vi "re_DataLog Write Number.vi"(0 "number":dbl format="%#_7g", 5 "time (current)":dbl=nan format="%<%H:%M:%S%2u\n%Y/%m/%d>T", 7 "tag":string, 9 "tag index in (use tag)":i32=-1, 11 "error in (no error)":errorcluster) -> (10 "tag index out":i32, 15 "error out":errorcluster)   [LabVIEW 2012]
doc: "Writes a number value to a tag. The current time is used as timestamp if no custom time is wired. The value is checked against any limit meta tags and coerced to any max/min meta tags. The current database must be live."
uses:
  typedefs/t_DataLog Tag Meta Tags Methods.ctl
  typedefs/clusters/t_DataLog Point.ctl
  typedefs/t_DataLog Tag Hash Methods.ctl
  luaview/typedefs/t_LuaVIEW Task List Methods.ctl
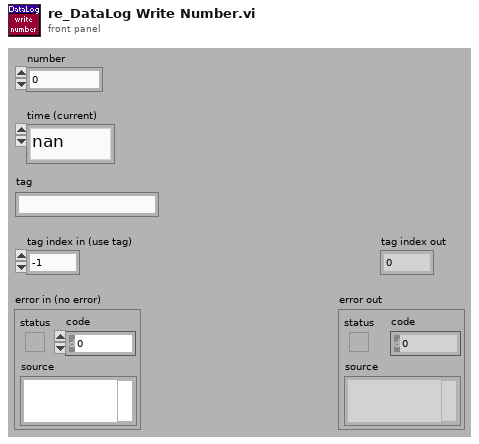
[diagram p1: front panel]
types:
  T1 = typedef "t_DataLog Point.ctl" = cluster{"time":dbl, "value":dbl}
  T2 = typedef "t_DataLog Tag Meta Tags Methods.ctl" = enum16{"initialize", "apply and write", "get exceeded", "get metas", "cleanup"}
  T3 = typedef "t_LuaVIEW Task List Methods.ctl" = enum16{"clear list", "add", "test", "remove", "get ref", "get task info", "get list", "get script info", "ongoing?", "resume", "pause", "stop", "confirm", "message"}
  T4 = typedef "t_DataLog Tag Hash Methods.ctl" = enum16{"initialize", "add tag", "index tag", "lookup", "#tags", "cleanup", "write recovery", "read recovery", "delete recovery"}
  T5 = typedef "et_DataLog Meta Tag Specifier.ctl" = enum32{"warn_lo", "warn_hi", "A_lo", "A_hi", "B_lo", "B_hi", "C_lo", "C_hi", "D_lo", "D_hi", "E_lo", "E_hi", "F_lo", "F_hi", "G_lo", "G_hi", "H_lo", "H_hi", "I_lo", "I_hi", "J_lo", "J_hi", "K_lo", "K_hi", "L_lo", "L_hi", "M_lo", "M_hi", "N_lo", "N_hi", "min", "max", "not a meta"}
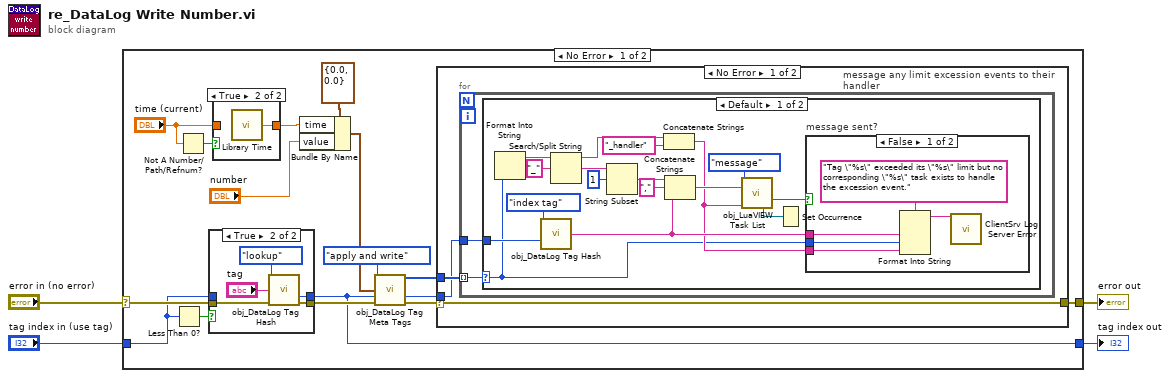
[diagram p0: block diagram]
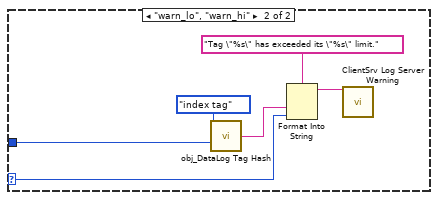
[diagram p4: hidden frame]
diagram:
  n1 = case shown="No Error" "error in (no error)" {
    selector: "error in (no error)" -> [w20 w65]
    tunnel: [w15 w65] -> w4
    tunnel: "tag index in (use tag)" -> [w6 w64]
    tunnel: [w5 w64] -> w1
    frame No Error {
      n2 = Less Than 0?(x=w6) -> (x < 0?=w19:bool)
      n3 = Not A Number/Path/Refnum?(number/path/refnum="time (current)") -> (NaN/Path/Refnum?=w12:bool)
      n4 = case shown="True" w19 {
        tunnel: w20 -> [w58 w63]
        tunnel: [w58 w61] -> w17
        tunnel: [w57 w60] -> w5
        tunnel: w6 -> [w57 _]
        frame False {
        }
        frame True {
          n5 = call "obj_DataLog Tag Hash.vi"("method"=t_DataLog_Tag_Hash_Methods."lookup", "tag in"="tag", "error in (no error)"=w63) -> ("tag index out"=w60:i32, "error out"=w61:errorcluster)  [unwired: 9 in, 2 out]
        }
      }
      n6 = case shown="True" w12 {
        tunnel: "time (current)" -> [w21 _]
        tunnel: [w21 w22] -> w10
        frame False {
        }
        frame True {
          n7 = call "Library Time.vi"() -> ("time"=w22:dbl)  [unwired: 1 in]
        }
      }
      n8 = Bundle By Name(cluster=T1 {"time"=0.0, "value"=0.0} ("point"), "time"=w10, "value"="number") -> (w7:T1)
      n9 = call "obj_DataLog Tag Meta Tags.vi"("method"=t_DataLog_Tag_Meta_Tags_Methods."apply and write", "point to write"=w7, "tag index in"=w5, "error in (no error)"=w17) -> ("limit events"=w14:T5[], "tag index dup"=w13:i32, "error out"=w16:errorcluster)  [unwired: 7 in, 2 out]
      n10 = case shown="No Error" w16 {
        selector: w16 -> [w23 w56]
        tunnel: [w23 w56] -> w15
        tunnel: w14 -> [w25 _]
        tunnel: w13 -> [w24 _]
        frame No Error {
          n11 = for "message any limit excession events to their handler" {
            tunnel: w25 -> [w26] mode=indexing
            tunnel: w24 -> [w27]
            n12 = case shown="Default" w26 {
              selector: w26 -> [w28 w51]
              tunnel: w27 -> [w35 w54]
              frame Default {
                n13 = Format Into String(w28) -> (resulting string=w44:string)  [unwired: 3 in, 1 out]
                n14 = call "obj_DataLog Tag Hash.vi"("method"=t_DataLog_Tag_Hash_Methods."index tag", "tag index in"=w35) -> ("tag out"=w31:string)  [unwired: 10 in, 3 out]
                n15 = Search/Split String(string=w44, search string/char (-)="_") -> (substring before match=w39:string, match + rest of string=w42:string)  [unwired: 1 in, 1 out]
                n16 = String Subset(string=w42, offset (0)=1) -> (substring=w40:string)  [unwired: 1 in]
                n17 = Concatenate Strings(w39, "_handler" ("string")) -> (w30:string)
                n18 = Concatenate Strings(w40, "," ("string"), w31) -> (w33:string)
                n19 = call "obj_LuaVIEW Task List.vi"("method"=t_LuaVIEW_Task_List_Methods."message", "message"=w33, "task identifier"=w30) -> ("set/ongoing"=w32:bool, "wakeup occurrence"=w29:refnum<k4>)  [unwired: 7 in, 4 out]
                n20 = Set Occurrence(w29) -> ()
                n21 = case "message sent?" shown="False" w32 {
                  tunnel: w28 -> [w48 _]
                  tunnel: w31 -> [w47 _]
                  tunnel: w30 -> [w46 _]
                  frame False {
                    n22 = Format Into String(format string="Tag \"%s\" exceeded its \"%s\" limit but no corresponding \"%s\" task exists to handle the excession event.", w47, w48, w46) -> (resulting string=w45:string)  [unwired: 2 in, 1 out]
                    n23 = call "ClientSrv Log Server Error.vi"("message (use cluster)"=w45) -> ()  [unwired: 15 in]
                  }
                  frame True {
                  }
                }
              }
              frame "warn_lo", "warn_hi" {
                n24 = call "obj_DataLog Tag Hash.vi"("method"=t_DataLog_Tag_Hash_Methods."index tag", "tag index in"=w54) -> ("tag out"=w52:string)  [unwired: 10 in, 3 out]
                n25 = Format Into String(format string="Tag \"%s\" has exceeded its \"%s\" limit.", w52, w51) -> (resulting string=w50:string)  [unwired: 2 in, 1 out]
                n26 = call "ClientSrv Log Server Warning.vi"("message (use cluster)"=w50) -> ()  [unwired: 15 in]
              }
            }
          }
        }
        frame Error {
        }
      }
    }
    frame Error {
    }
  }
  "error out" <- w4
  "tag index out" <- w1
